vi "set_last_minmax.vi"(4 "current_scen":u16, 5 "distance":dbl, 6 "min_vector":dbl[](array[numeric]), 7 "max_vector":dbl[](array[numeric]), 8 "array_in":T1(array[cluster])) -> (3 "array_out":T1(array[cluster]))   [LabVIEW 2011]
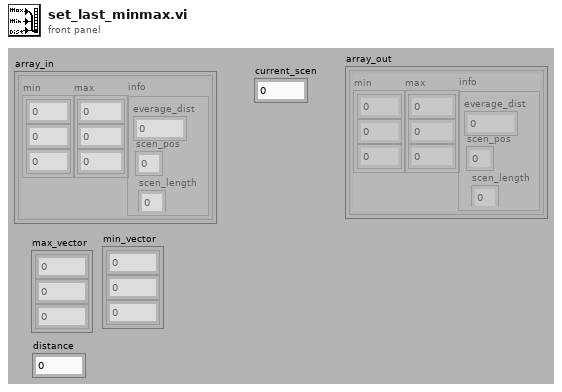
[diagram p1: front panel]
types:
  T1 = cluster{"min":dbl[], "max":dbl[], "info":cluster{"everage_dist":dbl, "scen_pos":u16, "scen_length":u16}}[]
  T2 = cluster{"min":dbl[], "max":dbl[], "info":cluster{"everage_dist":dbl, "scen_pos":u16, "scen_length":u16}}
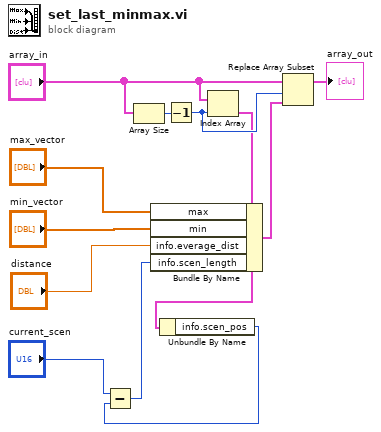
[diagram p0: block diagram]
diagram:
  n1 = Array Size(array="array_in") -> (size(s)=w9:i32)
  n2 = Decrement(x=w9) -> (x-1=w8:i32)
  n3 = Index Array(array="array_in", index=w8) -> (element=w3:T2)
  n4 = Unbundle By Name(w3) -> ("info.scen_pos"=w2:u16)
  n5 = Subtract(x="current_scen", y=w2) -> (x-y=w1:u16)
  n6 = Bundle By Name(cluster=w3, "max"="max_vector", "min"="min_vector", "info.everage_dist"="distance", "info.scen_length"=w1) -> (w12:T2)
  n7 = Replace Array Subset(array="array_in", new element=w12, index=w8) -> (→"array_out":T1)
